vi "Robot.Interface.GetJointRotation.vi"(8 "error in (no error)":errorcluster, 10 "JointType":enum16{"A_Shoulder", "B_Elbow", "C_Wrist"}(ring), 11 "Robot_Interface in":refnum<class "Robot_Interface.lvclass">) -> (0 "error out":errorcluster, 2 "Rotation (Deg)":dbl, 3 "Robot_Interface out":refnum<class "Robot_Interface.lvclass">)   [LabVIEW 2014]
uses:
  Robot_Interface.lvclass
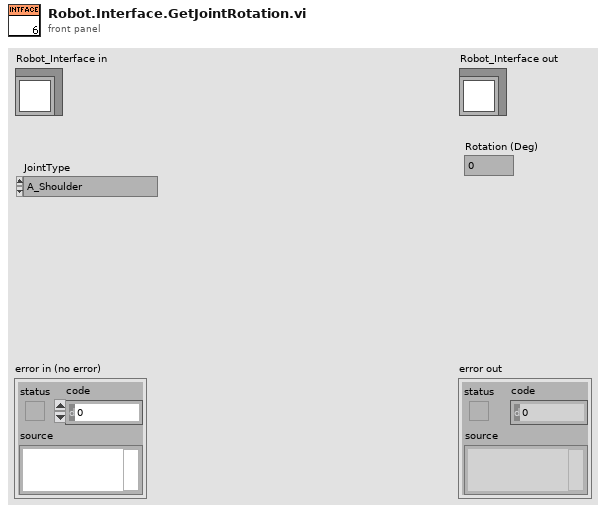
[diagram p1: front panel]
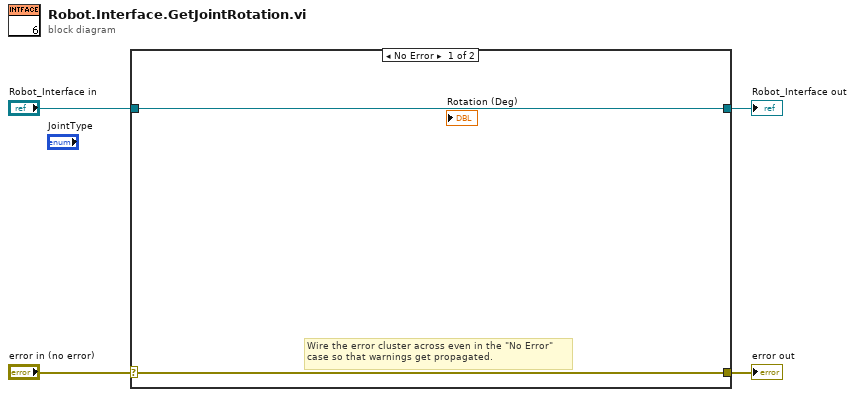
[diagram p0: block diagram]
diagram:
  n1 = case shown="No Error" "error in (no error)" {
    selector: "error in (no error)" -> [w5 w8]
    tunnel: [w5 w8] -> w3
    tunnel: [w6 w7] -> w1
    tunnel: "Robot_Interface in" -> [w6 w7]
    frame No Error {
      # "Wire the error cluster across even in the \"No Error\"\ncase so that warnings get propagated."
    }
    frame Error {
    }
  }
  "error out" <- w3
  "Robot_Interface out" <- w1
